vi "Synchio.PushPull.vi"(8 "error in (no error)":errorcluster, 10 "IO Info":T1={"AI task"=["", ""], "sampling info"={"Fs"=1000.0, "#s"=1000.0}, "AO Array"=[], "AO Task"=[], "Reset"=FALSE} {"sampling info"."Fs" format="%.2p"}, 11 "SynchIO.USB4431 in":refnum<class "SynchIO.USB4431.lvclass">) -> (0 "error out":errorcluster, 2 "Input Signals":waveform(dbl)[](array[waveform]), 3 "SynchIO.USB4431 out":refnum<class "SynchIO.USB4431.lvclass">)   [LabVIEW 2016, in "SynchIO.USB4431.lvclass"]
uses:
  SynchIO.USB4431.lvclass
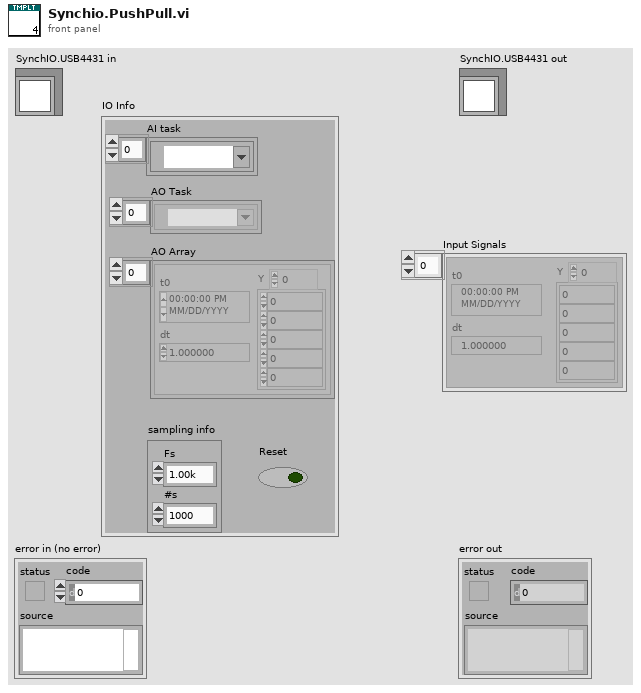
[diagram p1: front panel]
types:
  T1 = cluster{"AI task":refnum<k21>[], "sampling info":cluster{"Fs":dbl, "#s":dbl}, "AO Array":waveform(dbl)[], "AO Task":refnum<k21>[], "Reset":bool}
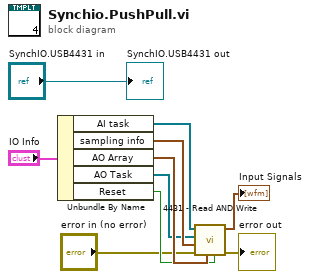
[diagram p0: block diagram]
diagram:
  n1 = Unbundle By Name("IO Info") -> ("AI task"=w10:refnum<k21>[], "sampling info"=w8:cluster{"Fs":dbl, "#s":dbl}, "AO Array"=w7:waveform(dbl)[], "AO Task"=w6:refnum<k21>[], "Reset"=w5:bool)
  n2 = call "4431 - Read AND Write.vi"("Reset"=w5, "AO Array"=w7, "error in (no error)"="error in (no error)", "sampling info"=w8, "AO Task"=w6, "AI task"=w10) -> ("error out"=→"error out":errorcluster, "Input Signals"=→"Input Signals":waveform(dbl)[])  [unwired: 4 in]
  "SynchIO.USB4431 out" <- "SynchIO.USB4431 in"
